vi "Exit In Place Element DVR.vi"(0 "Diagram in":refnum<vi>, 5 "Data Value":refnum<vi>, 7 "Outputs":refnum<vi>[](array[refnum]), 11 "error in (no error)":errorcluster) -> (4 "Diagram out":refnum<vi>, 6 "DVR":refnum<vi>, 8 "Outputs":refnum<vi>[](array[refnum]), 10 "DVR Error":refnum<vi>, 15 "error out":errorcluster)   [LabVIEW 2015, in "Scripting.lvlib"]
doc: "Exits the In Place Element Structure that owns <B>Diagram in</B>, supplying the structure's owning diagram at <B>Diagram out</B>.\n\n<B>Data Value</B> is the terminal to wire to the Write Data Value Reference node's data value terminal.\n\n<B>DVR</B> is the data value reference output terminal of the Write Data Value Reference node.\n\n<B>DVR Error</B> is the error output terminal of the Write Data Value Reference node."
uses:
  Scripting.lvlib
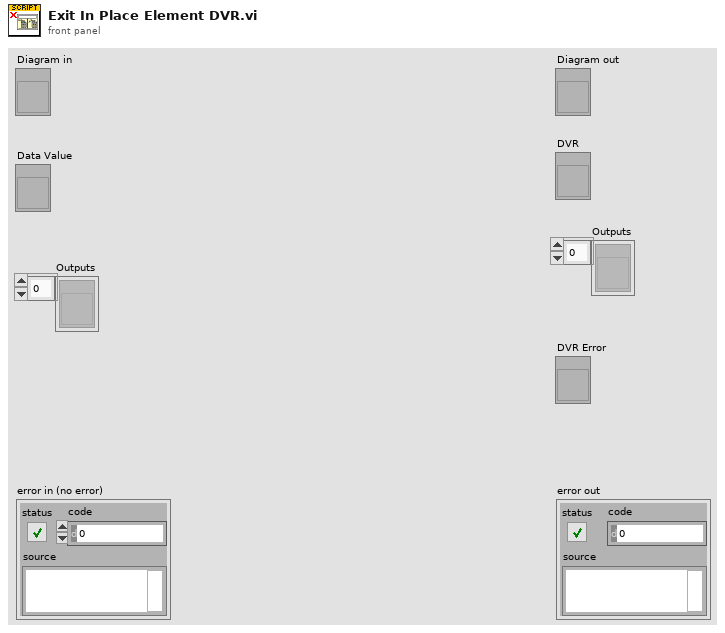
[diagram p1: front panel]
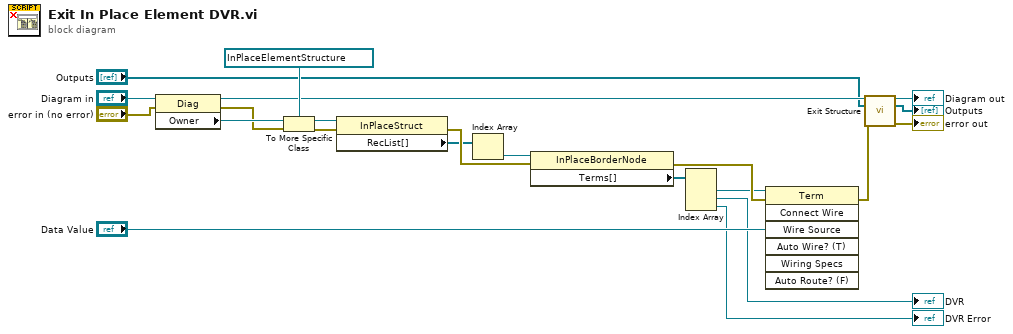
[diagram p0: block diagram]
diagram:
  n1 = property class="Diag"(reference="Diagram in", error in="error in (no error)") -> (reference out=w5:refnum<vi>, error out=w7:errorcluster, "Owner"=w20:refnum<vi>)
  n2 = To More Specific Class(target class=refnum<vi> refnum ("reference"), reference=w20, error in=w7) -> (specific class reference=w15:refnum<vi>, error out=w18:errorcluster)
  n3 = property class="InPlaceStruct"(reference=w15, error in=w18) -> (error out=w19:errorcluster, "RecList[]"=w16:refnum<vi>[])  [unwired: 1 out]
  n4 = Index Array(array=w16) -> (element=w17:refnum<vi>)  [unwired: 1 in]
  n5 = property class="InPlaceBorderNode"(reference=w17, error in=w19) -> (error out=w22:errorcluster, "Terms[]"=w13:refnum<vi>[])  [unwired: 1 out]
  n6 = Index Array(array=w13) -> (element #1=w21:refnum<vi>, element #2=→"DVR":refnum<vi>, element #3=→"DVR Error":refnum<vi>)  [unwired: 3 in]
  n7 = invoke class="Term" method="Connect Wire"(reference=w21, error in=w22, "Wire Source"="Data Value") -> (error out=w6:errorcluster)  [unwired: 4 in, 6 out]
  n8 = call "Exit Structure.vi"("Diagram in"=w5, "Outputs"="Outputs", "error in (no error)"=w6) -> ("Diagram out"=→"Diagram out":refnum<vi>, "Outputs"=→"Outputs":refnum<vi>[], "error out"=→"error out":errorcluster)  [unwired: 10 in]
